vi "Request New Connection.vi"(8 "error in (no error)":errorcluster, 10 "New Connection Request":refnum<class "INewConnectionCallback.lvclass">, 11 "Connection Factory Session In":refnum<data-value>) -> (0 "error out":errorcluster, 3 "Connection Factory Session Out":refnum<data-value>)   [LabVIEW 2019, in "ConnectionFactorySession.lvlib" / "ConnectionFactorySession.lvclass"]
uses:
  <vilib>/gpm_packages/@cs/Network-interface/Source/Connection Factory Session/ConnectionFactorySession/ConnectionFactorySession.lvclass
  <vilib>/gpm_packages/@cs/Network-interface/Source/Connection Factory Session/INewConnectionCallback/INewConnectionCallback.lvclass
  <vilib>/gpm_packages/@cs/Network-interface/Source/Connection Factory Session/ConnectionFactorySession/ConnectionFactorySession.lvclass/ConnectionFactorySession.ctl
  <vilib>/gpm_packages/@cs/Network-interface/Source/Connection Factory Session/Messages/Process Connection Msg/Process Connection Msg.lvclass/Process Connection Msg.ctl
  <vilib>/ActorFramework/Message Enqueuer/Message Enqueuer.lvclass/Message Enqueuer.ctl
  <vilib>/ActorFramework/Message Enqueuer/Enqueue.vi
  <vilib>/gpm_packages/@cs/Network-interface/Source/Connection Factory Session/Messages/Process Connection Msg/Process Connection Msg.lvclass
  C:/Program Files/National Instruments/LabVIEW 2019/vi.lib/ActorFramework/Message/Message.lvclass
  <vilib>/ActorFramework/Message Priority Queue/Priority Enqueue.vi
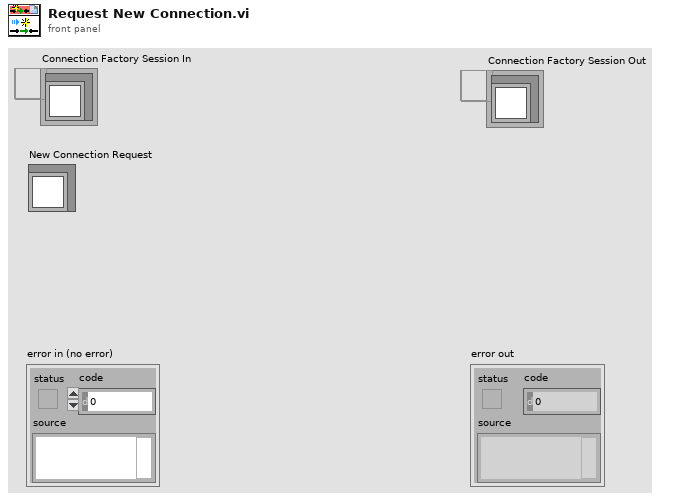
[diagram p1: front panel]
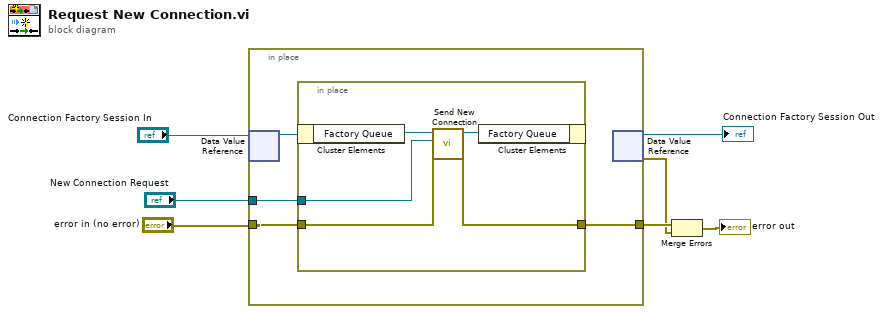
[diagram p0: block diagram]
diagram:
  n1 = in-place {
    in-place-border: "error in (no error)" -> [w10]
    in-place-border: [w9] -> w5
    in-place-border: "New Connection Request" -> [w8]
    n2 = in-place-dvr #1("Connection Factory Session In") -> (w11:refnum<class "ConnectionFactorySession.lvclass">)  [unwired: 1 out]
    n3 = in-place {
      in-place-border: w10 -> [w14]
      in-place-border: [w13] -> w9
      in-place-border: w8 -> [w12]
      n4 = in-place-cluster #2(w11) -> ("Factory Queue"=w16:refnum<class "Message Enqueuer.lvclass">)
      n5 = call <vilib>:"Send New Connection.vi"("error in (no error)"=w14, "New Connection Policy"=w12, "Message Enqueuer"=w16) -> ("error out"=w13:errorcluster, "Message Enqueuer out"=w15:refnum<class "Message Enqueuer.lvclass">)  [unwired: 7 in]
      n6 = in-place-cluster #2("Factory Queue"=w15) -> ()  [unwired: 1 out]
    }
    n7 = in-place-dvr #1() -> (→"Connection Factory Session Out":refnum<data-value>, w1:errorcluster)  [unwired: 1 in]
  }
  n8 = Merge Errors(w5, w1) -> (→"error out":errorcluster)
